vi "Close.vi"(8 "error in (no error)":errorcluster, 11 "APS7050 in":refnum<class "APS7050.lvclass">) -> (0 "error out":errorcluster, 3 "APS7050 out":refnum<class "APS7050.lvclass">)   [LabVIEW 2019, in "Concrete.lvlib" / "APS7050.lvclass"]
uses:
  APS7050.lvclass
  APS7050.lvclass/APS7050.ctl
  Harware Abstraction/Analog out/Analog out.lvclass
  <instrlib>/APS-7000 Series/APS-7000 Series.lvlib
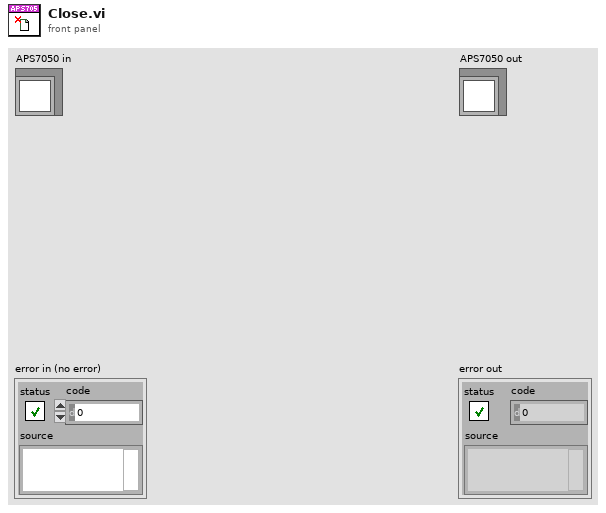
[diagram p1: front panel]
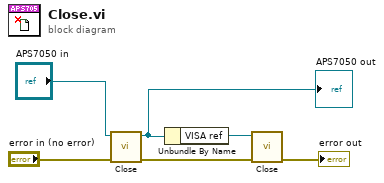
[diagram p0: block diagram]
diagram:
  n1 = call-parent <instrlib>:"Close.vi"("error in (no error)"="error in (no error)", "Instrument in"="APS7050 in") -> ("error out"=w3:errorcluster, "Instrument out"=w4:refnum<class "APS7050.lvclass">)  [unwired: 8 in]
  "APS7050 out" <- w4
  n2 = Unbundle By Name(w4) -> ("VISA ref"=w2:refnum<visa-resource-name>)
  n3 = call <instrlib>:"Close.vi"("error in (no error)"=w3, "VISA resource name"=w2) -> ("error out"=→"error out":errorcluster)  [unwired: 9 in]
